vi "sub_USRP_close_Tx.vi"(8 "Error in":errorcluster, 11 "Tx Session handle":refnum<k15>) -> (0 "Error out":errorcluster)   [LabVIEW 2012]
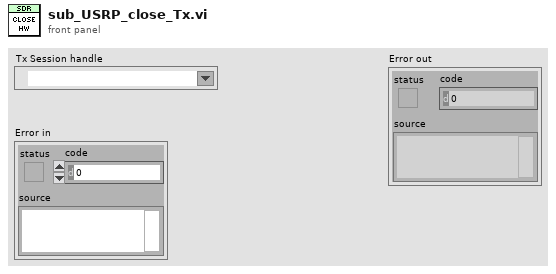
[diagram p1: front panel]
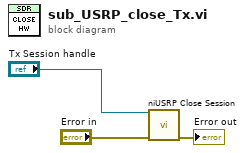
[diagram p0: block diagram]
diagram:
  n1 = call <instrlib>:"niUSRP Close Session.vi"("session handle"="Tx Session handle", "error in (no error)"="Error in") -> ("error out"=→"Error out":errorcluster)  [unwired: 13 in]
